vi "Check for Holding Register Mapping Conflicts.vi"(8 "error in (no error)":errorcluster, 11 "Group Ref in":T1 format="%.0x") -> (0 "error out":errorcluster, 1 "Conflicts?":bool, 2 "Conflicts":T2(array[cluster]), 3 "Coil Group Ref out":T1 format="%.0x")   [LabVIEW 2021, in "Modbus Master System Explorer.lvlib"]
uses:
  Modbus Master System Explorer.lvlib
  <vilib>/NI VeriStand/Custom Device API/Custom Device Item Ref.ctl
  Modbus Type.ctl
  <vilib>/NI VeriStand/Custom Device API/Custom Device API.lvlib
  Shared/Modbus Master Shared.lvlib
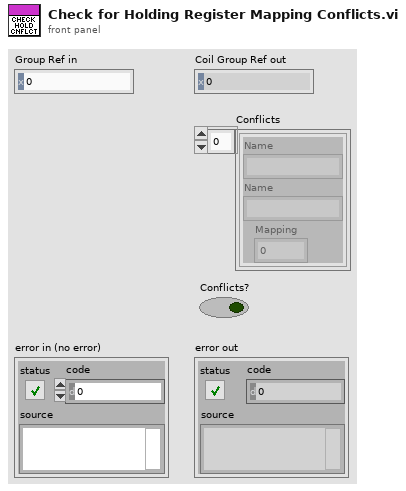
[diagram p1: front panel]
types:
  T1 = typedef "Custom Device API.lvlib/Custom Device Item Ref.ctl" = u64
  T2 = cluster{"Name":string, "Name":string, "Mapping":u16}[]
  T3 = typedef "Modbus Master Shared.lvlib/Modbus Type.ctl" = enum16{"Coil", "Discrete Input", "Holding Register", "Input Register"}
  T4 = typedef "Modbus Master Shared.lvlib/Mapping.ctl" = cluster{"DataType":T5, "Unit ID":u8, "Starting Address":u16, "Sub-Index (Bool)":u16, "VS Reference":T1}
  T5 = typedef "Modbus Master Shared.lvlib/DataType.ctl" = enum16{"Double", "Single", "I64", "I32", "I16", "I8", "U64", "U32", "U16", "U8", "Boolean"}
  T6 = typedef "Custom Device API.lvlib/Custom Device Item Info.ctl" = cluster{"Name":string, "Is Channel":bool, "GUID":string, "Is Waveform":bool}
  T7 = cluster{"Name":string, "Name":string, "Mapping":u16}
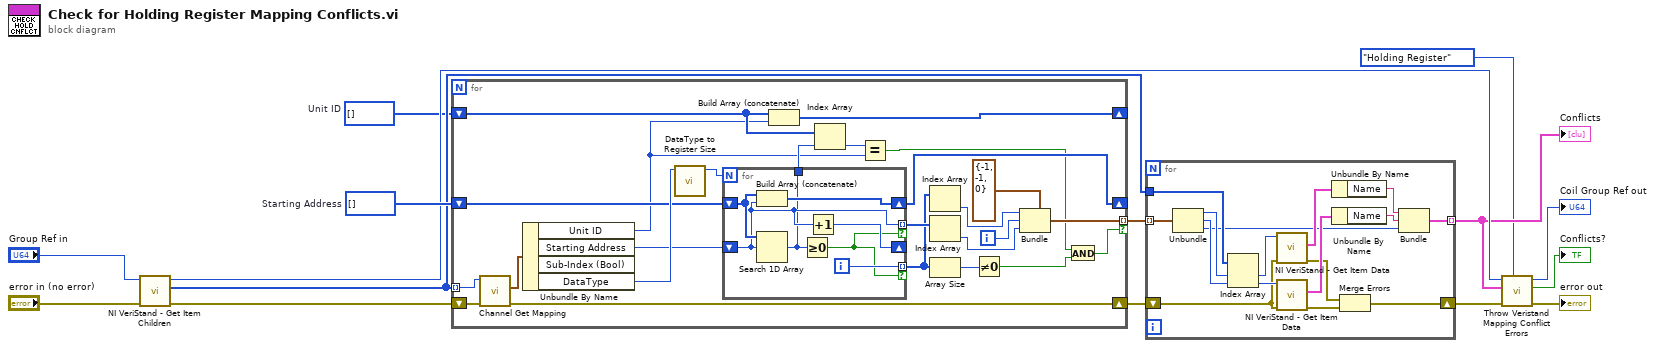
[diagram p0: block diagram]
diagram:
  w1 = u8[] []  # Unit ID
  w15 = u16[] []  # Starting Address
  n1 = call <vilib>:"NI VeriStand - Get Item Children.vi"("error in (no error)"="error in (no error)", "Item Ref in"="Group Ref in") -> ("error out"=w4:errorcluster, "Child Refs"=w5:T1[], "Item Ref out"=w11:T1)  [unwired: 6 in, 1 out]
  n2 = for {
    shift-right: [w33] -> _
    shift-left: w15 -> [w34]
    tunnel: [w39] -> w3 mode=indexing if=w16
    tunnel: w5 -> [w26] mode=indexing
    shift-right: [w24] -> w2
    shift-left: w4 -> [w25]
    shift-right: [w23] -> _
    shift-left: w1 -> [w21]
    i -> [w38]
    n3 = call "Channel Get Mapping.vi"("error in (no error)"=w25, "Item Ref in"=w26) -> ("error out"=w24:errorcluster, "Mapping"=w27:T4)  [unwired: 7 in, 1 out]
    n4 = Unbundle By Name(w27) -> ("Unit ID"=w19:u8, "Starting Address"=w35:u16, "DataType"=w37:T5)  [unwired: 1 out]
    n5 = call "DataType to Register Size.vi"("DataType"=w37) -> ("Registers"=w36:i32)  [unwired: 9 in, 1 out]
    n6 = for {
      N: w36 -> [_]
      shift-right: [w45] -> w33
      shift-left: w34 -> [w47]
      shift-right: [w46] -> _
      shift-left: w35 -> [w44]
      tunnel: [w43] -> w29 mode=indexing if=w42
      tunnel: [w44] -> w31 mode=indexing if=w42
      tunnel: [w41] -> w22
      i -> [w43]
      n7 = Build Array (concatenate)(w47, w44) -> (w45:u16[])
      n8 = Search 1D Array(1D array=w47, element=w44) -> (index of element=w41:i32)  [unwired: 1 in]
      n9 = Greater Or Equal To 0?(x=w41) -> (x >= 0?=w42:bool)
      n10 = Increment(x=w44) -> (x+1=w46:u16)
    }
    n11 = Build Array (concatenate)(w21, w19) -> (w23:u8[])
    n12 = Index Array(array=w21, index=w22) -> (element=w20:u8)
    n13 = Equal?(x=w20, y=w19) -> (x = y?=w18:bool)
    n14 = Index Array(array=w29) -> (element=w28:i32)  [unwired: 1 in]
    n15 = Index Array(array=w31) -> (element=w30:u16)  [unwired: 1 in]
    n16 = Array Size(array=w29) -> (size(s)=w32:i32)
    n17 = Not Equal To 0?(x=w32) -> (x != 0?=w17:bool)
    n18 = Bundle(cluster=cluster{"y":i32, "y 2":i32, "Mapping":u16} {"y"=-1, "y 2"=-1, "Mapping"=0} ("Conflicting Indices"), "y"=w28, "y 2"=w38, "Mapping"=w30) -> (w39:cluster{"y":i32, "y 2":i32, "Mapping":u16})
    n19 = And(x=w18, y=w17) -> (x .and. y?=w16:bool)
  }
  n20 = for {
    tunnel: w3 -> [w63] mode=indexing
    tunnel: w5 -> [w62]
    tunnel: [w53] -> w10 mode=indexing
    shift-right: [w48] -> w9
    shift-left: w2 -> [w51]
    n21 = Unbundle(w63) -> ("y"=w61:i32, "y 2"=w60:i32, "Mapping"=w52:u16)
    n22 = Index Array(array=w62, index #1=w61, index #2=w60) -> (element #1=w59:T1, element #2=w58:T1)
    n23 = call <vilib>:"NI VeriStand - Get Item Data.vi"("error in (no error)"=w51, "Item Ref in"=w59) -> ("error out"=w50:errorcluster, "Item Info"=w57:T6)  [unwired: 8 out]
    n24 = call <vilib>:"NI VeriStand - Get Item Data.vi"("error in (no error)"=w51, "Item Ref in"=w58) -> ("error out"=w49:errorcluster, "Item Info"=w56:T6)  [unwired: 8 out]
    n25 = Unbundle By Name(w57) -> ("Name"=w55:string)
    n26 = Unbundle By Name(w56) -> ("Name"=w54:string)
    n27 = Merge Errors(w50, w49) -> (w48:errorcluster)
    n28 = Bundle("Name"=w55, "Name"=w54, "Mapping"=w52) -> (w53:T7)  [unwired: 1 in]
  }
  "Conflicts" <- w10
  n29 = call "Throw Veristand Mapping Conflict Errors.vi"("Type"=Modbus_Type."Holding Register", "error in (no error)"=w9, "Conflicts In"=w10, "Item Ref in"=w11) -> ("error out"=→"error out":errorcluster, "Conflicts?"=→"Conflicts?":bool, "Node Ref out"=→"Coil Group Ref out":T1)  [unwired: 5 in]
